vi "Launcher.vi"() -> ()   [LabVIEW 2020]
uses:
  Simple UI/Simple UI/Simple UI.lvclass
  C:/Program Files (x86)/National Instruments/LabVIEW 2020/vi.lib/ActorFramework/Actor/Actor.lvclass
  <vilib>/ActorFramework/Actor/Actor.lvclass
panel:
  out "error out":errorcluster
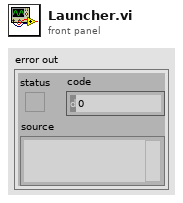
[diagram p1: front panel]
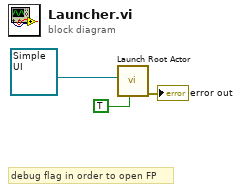
[diagram p0: block diagram]
diagram:
  # "debug flag in order to open FP"
  n1 = call <vilib>:"Launch Root Actor.vi"("Open Actor Core front panel? (F)"=TRUE, "Actor"=refnum<class "Simple UI.lvclass"> refnum ("Simple UI.lvlib:Simple UI.lvclass")) -> ("error out"=→"error out":errorcluster)  [unwired: 8 in, 1 out]
